vi "Launch a File with its Default Application.vi"(8 "error in (no error)":errorcluster caption="错误输入（无错误）", 11 "File Path":path) -> (0 "error out":errorcluster caption="错误输出")   [LabVIEW 2011]
panel:
  # "用默认程序打开文件"
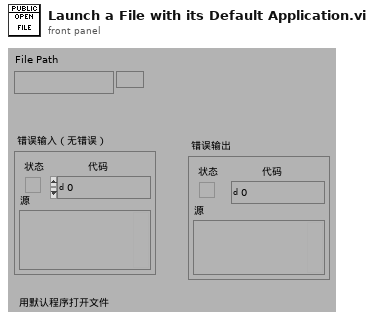
[diagram p1: front panel]
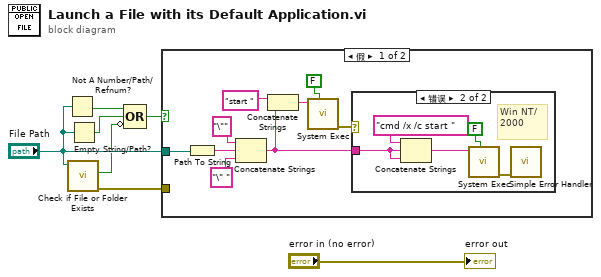
[diagram p0: block diagram]
diagram:
  n1 = Not A Number/Path/Refnum?(number/path/refnum="File Path") -> (NaN/Path/Refnum?=w5:bool)
  n2 = call <vilib>:"Check if File or Folder Exists.vi"("path"="File Path") -> ("error out"=w1:errorcluster, "file or folder exists?"=w3:bool)  [unwired: 8 in, 1 out]
  n3 = Empty String/Path?(string/path="File Path") -> (empty?=w4:bool)
  n4 = Compound Arithmetic op=OR(w5, w4, invert w3) -> (w2:bool)
  n5 = case shown="假" w2 {
    tunnel: "File Path" -> [w8 _]
    tunnel: w1 -> [_ _]
    frame False {
      n6 = Path To String(path=w8) -> (string=w9:string)
      n7 = Concatenate Strings("\"" ("Substring"), w9, "\" " ("Substring")) -> (w11:string)
      n8 = Concatenate Strings("start " ("Substring"), w11) -> (w12:string)
      n9 = call <vilib>:"System Exec.vi"("wait until completion? (T)"=FALSE ("Wait until done"), "command line"=w12) -> ("error out"=w13:errorcluster)  [unwired: 6 in, 3 out]
      n10 = case shown="错误" w13 {
        tunnel: w11 -> [_ w17]
        frame No Error {
          # "Win 95/98/Me"
        }
        frame Error {
          # "Win NT/\n2000"
          n11 = Concatenate Strings("cmd /x /c start ", w17, w17) -> (w19:string)
          n12 = call <vilib>:"System Exec.vi"("wait until completion? (T)"=FALSE ("Wait until done"), "command line"=w19) -> ("error out"=w18:errorcluster)  [unwired: 6 in, 3 out]
          n13 = call <vilib>:"Simple Error Handler.vi"("error in (no error)"=w18) -> ()  [unwired: 4 in, 5 out]
        }
      }
    }
    frame True {
    }
  }
  "error out" <- "error in (no error)"
